vi "非模式对话框.vi"() -> (3 "Cancelled?":bool caption="取消？")   [LabVIEW 2013]
doc: "该模板用于创建能够进行事件处理的对话框。"
panel:
  out "VI名称":string
  out "VI路径":path
  out "VI类型":T1(ring)
  in  "Cancel":bool caption="取消"
  in  "OK":bool caption="确定"
  # "1、打开VI属性对话框。\n2、在外观选项中，先设置为“对话框”，然后再设置为“自定义”。\n3、在窗口动作中，选择“默认”"
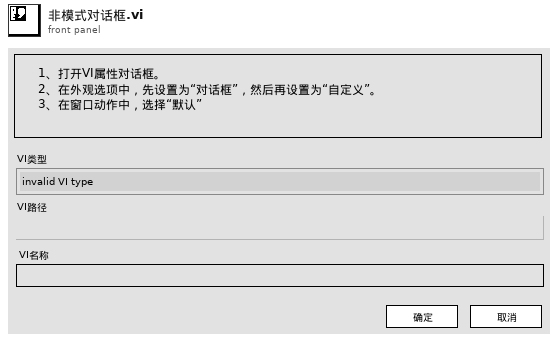
[diagram p1: front panel]
types:
  T1 = enum32{"invalid VI type", "Standard VI", "Control VI", "Global VI", "Polymorphic VI", "Configuration VI", "SubSystem", "Facade VI", "Method VI", "Statechart Diagram VI"}
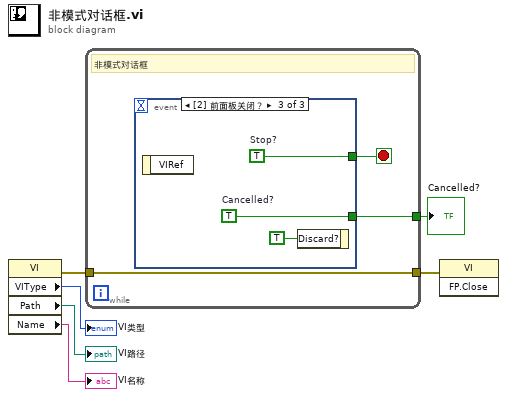
[diagram p0: block diagram]
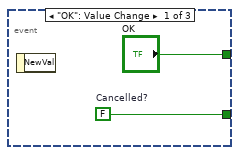
[diagram p2: hidden frame]
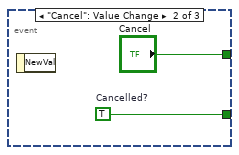
[diagram p3: hidden frame]
diagram:
  n1 = property class="VI"() -> (error out=w2:errorcluster, "VIType"=→"VI类型":T1, "Path"=→"VI路径":path, "Name"=→"VI名称":string)  [unwired: 2 in, 1 out]
  n2 = while {
    tunnel: [w8] -> w6
    tunnel: w2 -> [w7]
    tunnel: [w7] -> w1
    stop <- w9 stop-if-true
    # "非模式对话框"
    n3 = event shown="[2] 前面板关闭？" {
      selector: _ -> [_ _ _]
      dyn-events: _ -> [_ _ _]
      timeout: _ -> [_ _ _]
      tunnel: ["OK" "Cancel" w15] -> w9
      tunnel: [w11 w13 w14] -> w8
      event "OK": Value Change {
        w11 = FALSE  # Cancelled?
        n4 = event-data() -> ()  [unwired: 1 in, 1 out]
      }
      event "Cancel": Value Change {
        w13 = TRUE  # Cancelled?
        n5 = event-data() -> ()  [unwired: 1 in, 1 out]
      }
      event Panel Close? {
        w14 = TRUE  # Cancelled?
        w15 = TRUE  # Stop?
        n6 = event-data() -> ()  [unwired: 1 in, 1 out]
        n7 = event-data("Discard?"=TRUE) -> ()  [unwired: 1 in, 1 out]
      }
    }
  }
  "Cancelled?" <- w6
  n8 = invoke class="VI" method="FP.Close"(error in=w1) -> ()  [unwired: 2 in, 3 out]
